vi "sleep_detection_low_mobility.vi"(8 "Deprivation\nparameters":T1={"Frame Row"=0, "Kstd"=40.0, "# Images for\nsleep detection"=10, "Kmean"=1.5, "Start time of sleep detection"=1000, 0, "Max deprivation length"=3600, "Max # TTL"=10000, "Delay detection start by x images after first detection"=0, "Minimum Interval between TTL pulses"=0, "Delay sleep detection\nby x detections"=9, "# Total immobility\n detections"=0.0, "Pause max # adjacent\nTTL"=0, "TTL x start\ntime deprivation\n"=0.0, "Max #\nadjacent TTL"=10000, " Ca2+\nmode"=0} {"?" items=["1", "2", "3", "4"]; "Frame Row" items=["1", "2", "3", "4"]}, 10 "Global image \nsubtraction array":dbl[](array[numeric]), 11 "Local image \nsubtraction array":dbl[](array[numeric])) -> (3 "Sleep detection":bool)   [LabVIEW 2011]
uses:
  <vilib>/Analysis/baseanly.llb/Std Deviation and Variance.vi
  <vilib>/Analysis/NI_AALBase.lvlib
panel:
  # "Sleep deprivation settings"
  # "Select deprivation animal"
  # "Deprive image in row"
  # "Deprive image in column"
  # "Sleep detection parameters"
  # "Sleep deprivation parameters"
  # "Delay deprivation start:"
  # "Pause deprivation (images):"
  # "Stop deprivation after:"
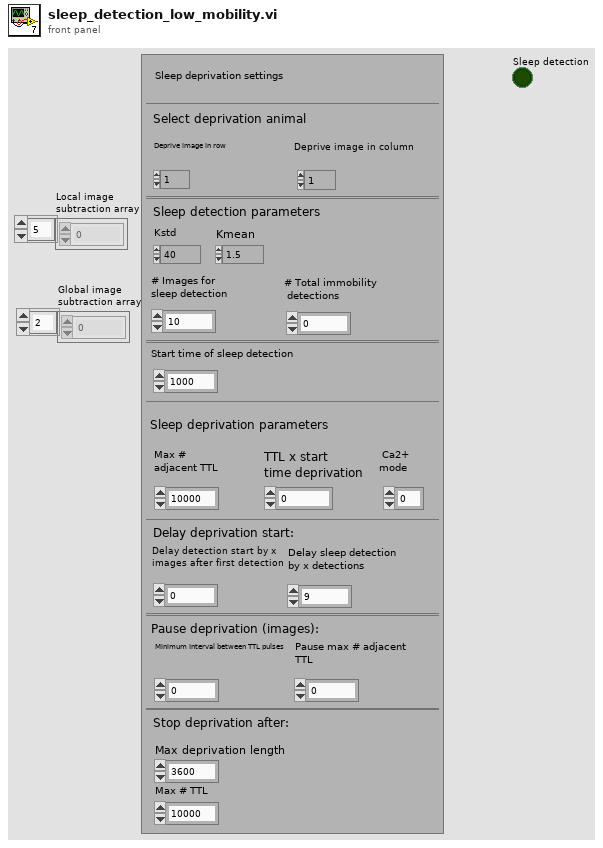
[diagram p1: front panel]
types:
  T1 = cluster{"Frame Row":u32, "Kstd":dbl, "# Images for\nsleep detection":i32, "Kmean":dbl, "Start time of sleep detection":i32, u32, "Max deprivation length":i32, "Max # TTL":i32, "Delay detection start by x images after first detection":i32, "Minimum Interval between TTL pulses":i32, "Delay sleep detection\nby x detections":i32, "# Total immobility\n detections":dbl, "Pause max # adjacent\nTTL":i32, "TTL x start\ntime deprivation\n":dbl, "Max #\nadjacent TTL":i32, " Ca2+\nmode":i32}
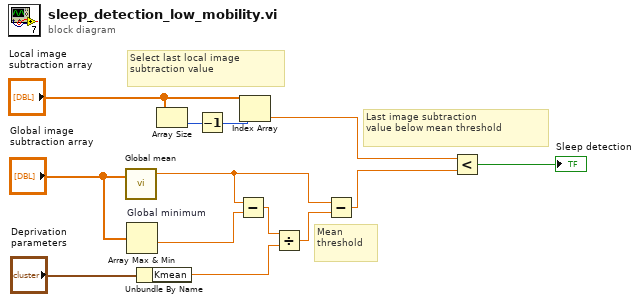
[diagram p0: block diagram]
diagram:
  # "Mean \nthreshold"
  # "Last image subtraction\nvalue below mean threshold"
  # "Select last local image \nsubtraction value"
  n1 = call "Global mean"("X"="Global image \nsubtraction array") -> ("mean"=w8:dbl)  [unwired: 1 in, 2 out]
  n2 = Array Max & Min "Global minimum"(array="Global image \nsubtraction array") -> (min value=w13:dbl)  [unwired: 3 out]
  n3 = Unbundle By Name("Deprivation\nparameters") -> ("Kmean"=w5:dbl)
  n4 = Array Size(array="Local image \nsubtraction array") -> (size(s)=w11:i32)
  n5 = Decrement(x=w11) -> (x-1=w9:i32)
  n6 = Subtract(x=w8, y=w13) -> (x-y=w12:dbl)
  n7 = Index Array(array="Local image \nsubtraction array", index=w9) -> (element=w10:dbl)
  n8 = Divide(x=w12, y=w5) -> (x/y=w7:dbl)
  n9 = Subtract(x=w8, y=w7) -> (x-y=w6:dbl)
  n10 = Less?(x=w10, y=w6) -> (x < y?=→"Sleep detection":bool)
